vi "Build Control Tree.vi"(8 "error in (no error)":errorcluster, 11 "Control List in":refnum<class "Control List.lvclass">) -> (0 "error out":errorcluster, 2 "Control Tree":refnum<class "Tree Map.lvclass">, 3 "Control List out":refnum<class "Control List.lvclass">)   [LabVIEW 2020, in "VolatusGUIEditor.lvlib" / "Control List.lvclass"]
uses:
  Control List.lvclass
  lv-tree-tools/Tree Map/Tree Map/Tree Map.lvclass
  Control List.lvclass/Control List.ctl
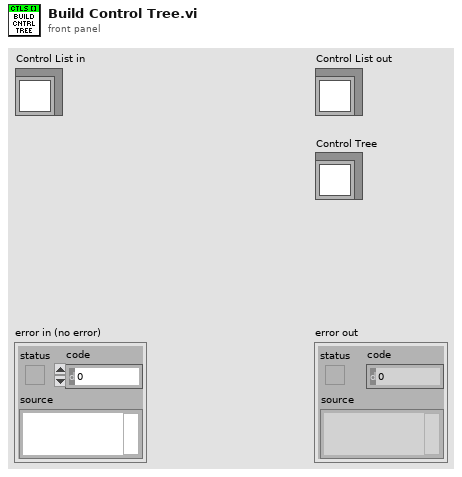
[diagram p1: front panel]
types:
  T1 = typedef "VolatusGUIEditor.lvlib/Control Info.ctl" = cluster{"Description":string, "Hierarchy":string[], "Image":T2, "Element Type":string}
  T2 = typedef "imagedata.ctl" = cluster{"image type":i32, "image depth":i32, "image":u8[], "mask":u8[], "colors":u32[], "Rectangle":cluster{"left":i16, "top":i16, "right":i16, "bottom":i16}}
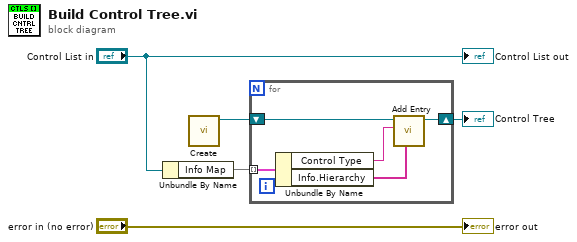
[diagram p0: block diagram]
diagram:
  n1 = Unbundle By Name("Control List in") -> ("Info Map"=w3:map{string, T1})
  n2 = call "Create.vi"() -> ("Tree Map out"=w2:refnum<class "Tree Map.lvclass">)  [unwired: 10 in, 1 out]
  n3 = for {
    tunnel: w3 -> [w10] mode=indexing
    shift-right: [w6] -> w1
    shift-left: w2 -> [w9]
    n4 = Unbundle By Name(w10) -> ("Control Type"=w8:string, "Info.Hierarchy"=w7:string[])
    n5 = call "Add Entry.vi"("Parent (None)"=w7, "Name"=w8, "Tree Map in"=w9) -> ("Tree Map out"=w6:refnum<class "Tree Map.lvclass">)  [unwired: 6 in, 2 out]
  }
  "Control Tree" <- w1
  "error out" <- "error in (no error)"
  "Control List out" <- "Control List in"
